vi "optionsAcq_channel_gainIndex.vi"(8 "error in (no error)":errorcluster, 9 "readWrite":enum16{"read", "write"}(ring), 10 "gainIndex":u16, 11 "OSAchannel in":refnum<class "OSAchannel.lvclass">) -> (0 "error out":errorcluster, 1 "status_ftsLib":i32, 2 "gainLevel":i32, 3 "OSAchannel out":refnum<class "OSAchannel.lvclass">)   [LabVIEW 2010, in "OSAchannel.lvclass"]
uses:
  OSAchannel.lvclass
  OSAchannel.lvclass/OSAchannel.ctl
  OSA20X_misc.lvlib
  _dll/LVLib/FTSLib.lvlib
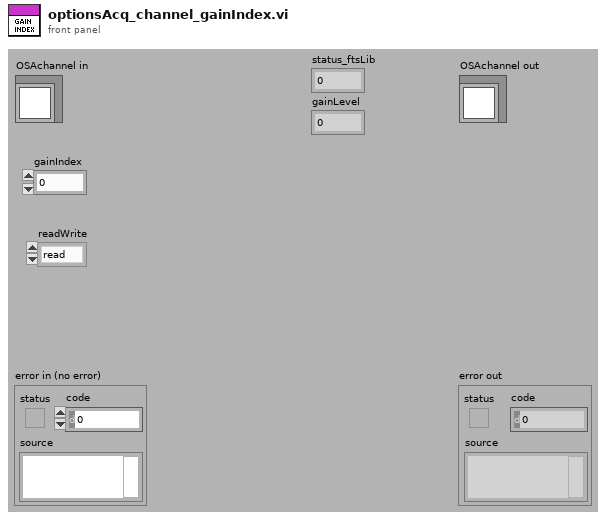
[diagram p1: front panel]
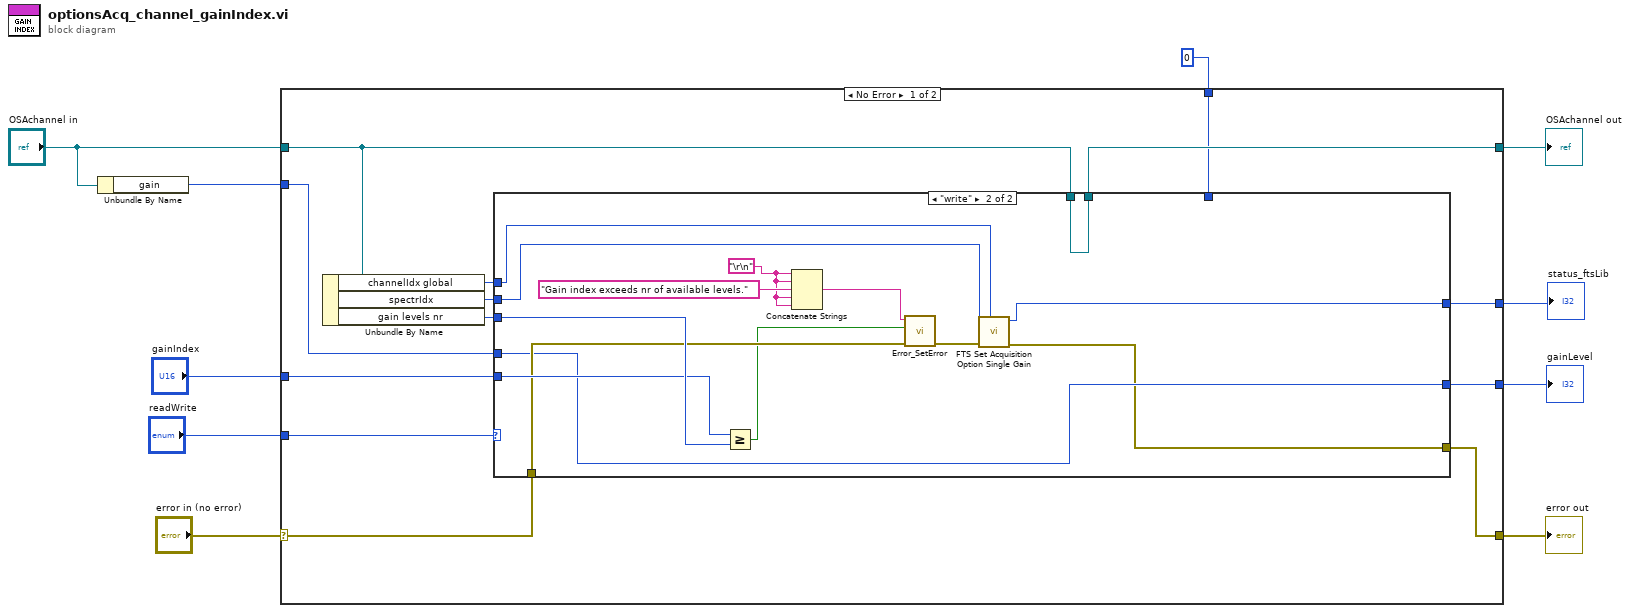
[diagram p0: block diagram]
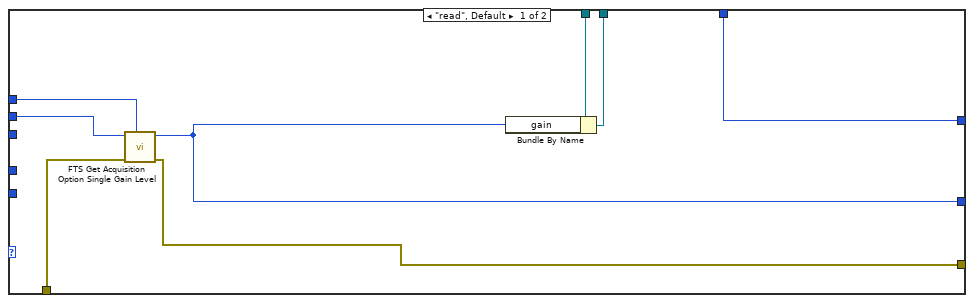
[diagram p2: hidden frame]
diagram:
  n1 = Unbundle By Name("OSAchannel in") -> ("gain"=w1:i32)
  n2 = case shown="No Error" "error in (no error)" {
    selector: "error in (no error)" -> [w16 w49]
    tunnel: [w14 w49] -> w9
    tunnel: [w18 w48] -> w8
    tunnel: "OSAchannel in" -> [w19 w48]
    tunnel: "gainIndex" -> [w22 _]
    tunnel: "readWrite" -> [w21 _]
    tunnel: [w20 w47] -> w5
    tunnel: 0 ("status") -> [w17 w47]
    tunnel: [w13 w46] -> w3
    tunnel: w1 -> [w12 w46]
    frame No Error {
      n3 = Unbundle By Name(w19) -> ("channelIdx global"=w11:u16, "spectrIdx"=w23:u16, "gain levels nr"=w15:u16)
      n4 = case shown="\"write\"" w21 {
        tunnel: w23 -> [w26 w35]
        tunnel: [w29 w32] -> w20
        tunnel: [w24 w33] -> w14
        tunnel: w22 -> [_ w43]
        tunnel: w19 -> [w31 w45]
        tunnel: [w30 w45] -> w18
        tunnel: w17 -> [w29 _]
        tunnel: w16 -> [w25 w42]
        tunnel: w15 -> [_ w44]
        tunnel: [w28 w37] -> w13
        tunnel: w12 -> [_ w37]
        tunnel: w11 -> [w27 w34]
        frame "read", Default {
          n5 = call "FTS Get Acquisition Option Single Gain Level.vi"("channel"=w27, "error in (no error)"=w25, "specIndex"=w26) -> ("error out"=w24:errorcluster, "function return"=w28:i32)  [unwired: 7 in]
          n6 = Bundle By Name(cluster=w31, "gain"=w28) -> (w30:refnum<class "OSAchannel.lvclass">)
        }
        frame "write" {
          w38 = "\r\n"
          n7 = Greater Or Equal?(x=w43, y=w44) -> (x >= y?=w39:bool)
          n8 = Concatenate Strings(w38, w38, "Gain index exceeds nr of available levels." ("source(\"\")"), w38, w38) -> (w40:string)
          n9 = call "Error_SetError.vi"("error in"=w42, "status (true)"=w39, "source(\"\")"=w40) -> ("error out"=w36:errorcluster)  [unwired: 4 in]
          n10 = call "FTS Set Acquisition Option Single Gain.vi"("channel"=w34, "error in (no error)"=w36, "specIndex"=w35) -> ("error out"=w33:errorcluster, "function return"=w32:i32)  [unwired: 7 in]
        }
      }
    }
    frame Error {
    }
  }
  "error out" <- w9
  "OSAchannel out" <- w8
  "status_ftsLib" <- w5
  "gainLevel" <- w3
